vi "Lock_in_calculation.vi"(8 "Sin_Cos_Scale":fxp<+/-,16,2>, 11 "Input Data":u64[](array[numeric])) -> (0 "Phase":dbl, 3 "Amplitude":dbl)   [LabVIEW 2018]
uses:
  <vilib>/Analysis/baseanly.llb/Mean (DBL).vi
  <vilib>/Analysis/NI_AALBase.lvlib
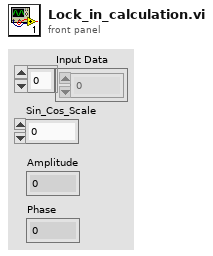
[diagram p1: front panel]
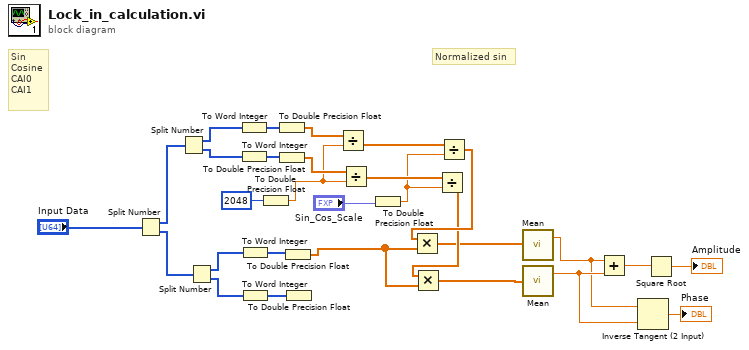
[diagram p0: block diagram]
diagram:
  # "Normalized sin"
  # "Sin\nCosine\nCAI0\nCAI1"
  n1 = Split Number(x="Input Data") -> (hi(x)=w28:u32[], lo(x)=w27:u32[])
  n2 = Split Number(x=w28) -> (hi(x)=w26:u16[], lo(x)=w25:u16[])
  n3 = Split Number(x=w27) -> (hi(x)=w24:u16[], lo(x)=w23:u16[])
  n4 = To Word Integer(number=w26) -> (16bit integer=w22:i16[])
  n5 = To Word Integer(number=w25) -> (16bit integer=w21:i16[])
  n6 = To Word Integer(number=w24) -> (16bit integer=w12:i16[])
  n7 = To Word Integer(number=w23) -> (16bit integer=w11:i16[])
  n8 = To Double Precision Float(number=2048) -> (double precision float=w18:dbl)
  n9 = To Double Precision Float(number=w22) -> (double precision float=w19:dbl[])
  n10 = To Double Precision Float(number=w21) -> (double precision float=w20:dbl[])
  n11 = To Double Precision Float(number=w12) -> (double precision float=w8:dbl[])
  n12 = To Double Precision Float(number=w11) -> ()  [unwired: 1 out]
  n13 = Divide(x=w19, y=w18) -> (x/y=w14:dbl[])
  n14 = Divide(x=w20, y=w18) -> (x/y=w15:dbl[])
  n15 = To Double Precision Float(number="Sin_Cos_Scale") -> (double precision float=w13:dbl)
  n16 = Divide(x=w15, y=w13) -> (x/y=w9:dbl[])
  n17 = Multiply(x=w9, y=w8) -> (x*y=w6:dbl[])
  n18 = Divide(x=w14, y=w13) -> (x/y=w10:dbl[])
  n19 = Multiply(x=w10, y=w8) -> (x*y=w7:dbl[])
  n20 = call-poly <vilib>:"Mean.vi"("X"=w7) -> ("mean"=w3:dbl)  [unwired: 1 out]
  n21 = call-poly <vilib>:"Mean.vi"("X"=w6) -> ("mean"=w4:dbl)  [unwired: 1 out]
  n22 = Add(x=w3, y=w4) -> (x+y=w5:dbl)
  n23 = Inverse Tangent (2 Input)(1:w4, 2:w3) -> (0:→"Phase":dbl)
  n24 = Square Root(x=w5) -> (sqrt(x)=→"Amplitude":dbl)
